vi "niRFUtil RFHS Channelizer FineTuneResamplerCheck CSG.vi"(0 "fs [Hz]":dbl=1.0 format="%#_6p", 5 "fs shift (ppm)":dbl format="%#_6p", 7 "phase shift (samples)":dbl, 11 "error in (no error)":errorcluster) -> (15 "error out":errorcluster)   [LabVIEW 2015, in "niRFUtil.lvlib"]
uses:
  niRFUtil.lvlib
  Includes/niRFUtil RFHS Channelizer ChannelizerErrors.ctl
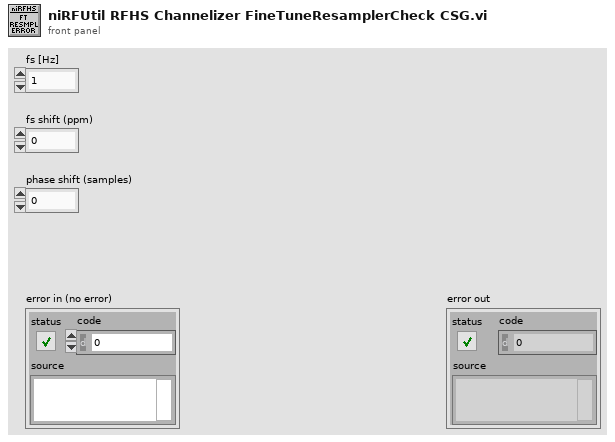
[diagram p1: front panel]
types:
  T1 = typedef "niRFUtil.lvlib/niRFUtil RFHS Channelizer ChannelizerErrors.ctl" = enum32{"No Error", "Invalid Channel", "Internal Error", "Invalid Channel fs", "Invalid Phase Shift", "Invalid fs", "Invalid Number Of Channles", "Invalid FFT Channel fs", "Invalid Resampler Channel fs", "Not a 15kHz Multiple", "Invalid Channel fc", "Invalid passBW/stopBW", "Coerced Rejection", "Requires Internal Buffer", "Duplicated Destination Channel Name", "Configuration Format Error", "Illegal Execution state", "DLL not found", "DLL loading failure", "AVX instruction failure"}
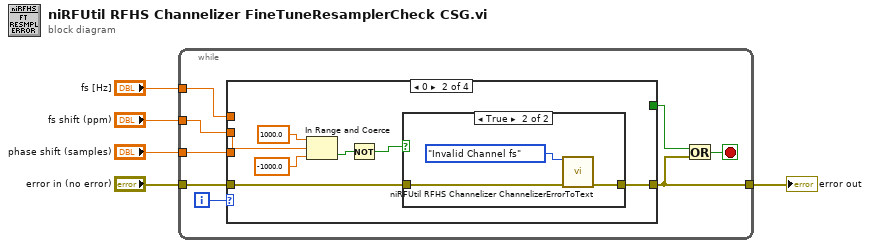
[diagram p0: block diagram]
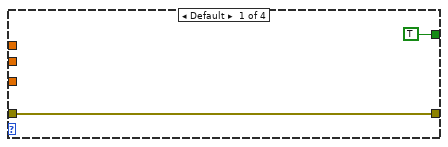
[diagram p2: hidden frame]
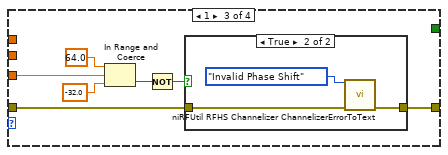
[diagram p4: hidden frame]
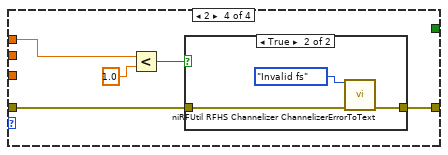
[diagram p6: hidden frame]
diagram:
  n1 = while {
    tunnel: "error in (no error)" -> [w13]
    tunnel: [w6] -> w3
    tunnel: "fs shift (ppm)" -> [w10]
    tunnel: "phase shift (samples)" -> [w9]
    tunnel: "fs [Hz]" -> [w8]
    i -> [w11]
    stop <- w12 stop-if-true
    n2 = case shown="0" w11 {
      tunnel: [TRUE _ _ _] -> w7
      tunnel: w13 -> [w14 w22 w33 w42]
      tunnel: [w14 w21 w32 w41] -> w6
      tunnel: w10 -> [_ w16 _ _]
      tunnel: w9 -> [_ _ w28 _]
      tunnel: w8 -> [_ _ _ w40]
      frame Default {
      }
      frame 0 {
        n3 = In Range and Coerce(upper limit=1000.0, x=w16, lower limit=-1000.0) -> (In Range?=w18:bool)  [unwired: 1 out]
        n4 = Not(x=w18) -> (.not. x?=w17:bool)
        n5 = case shown="True" w17 {
          tunnel: w22 -> [w23 w26]
          tunnel: [w23 w24] -> w21
          frame False {
          }
          frame True {
            n6 = call "niRFUtil RFHS Channelizer ChannelizerErrorToText.vi"("Error List"=niRFUtil_RFHS_Channelizer_ChannelizerErrors."Invalid Channel fs", "error in (no error)"=w26) -> ("error out"=w24:errorcluster)  [unwired: 13 in]
          }
        }
      }
      frame 1 {
        n7 = In Range and Coerce(upper limit=64.0, x=w28, lower limit=-32.0) -> (In Range?=w30:bool)  [unwired: 1 out]
        n8 = Not(x=w30) -> (.not. x?=w29:bool)
        n9 = case shown="True" w29 {
          tunnel: w33 -> [w34 w37]
          tunnel: [w34 w35] -> w32
          frame False {
          }
          frame True {
            n10 = call "niRFUtil RFHS Channelizer ChannelizerErrorToText.vi"("Error List"=niRFUtil_RFHS_Channelizer_ChannelizerErrors."Invalid Phase Shift", "error in (no error)"=w37) -> ("error out"=w35:errorcluster)  [unwired: 13 in]
          }
        }
      }
      frame 2 {
        n11 = Less?(x=w40, y=1.0) -> (x < y?=w38:bool)
        n12 = case shown="True" w38 {
          tunnel: w42 -> [w43 w46]
          tunnel: [w43 w44] -> w41
          frame False {
          }
          frame True {
            n13 = call "niRFUtil RFHS Channelizer ChannelizerErrorToText.vi"("Error List"=niRFUtil_RFHS_Channelizer_ChannelizerErrors."Invalid fs", "error in (no error)"=w46) -> ("error out"=w44:errorcluster)  [unwired: 13 in]
          }
        }
      }
    }
    n14 = Or(x=w7, y=w6) -> (x .or. y?=w12:bool)
  }
  "error out" <- w3
